vi "LSMcontroller_v63_3Dfocus.vi"() -> ()   [LabVIEW 2015] (continued)
                    n3624 = call "2pparameters.vi"("Params in"=w485, "command"="set") -> ()  [unwired: 1 out]
                  }
                }
              }
            }
          }
          event "Add DO wave": Value Change {
            n3625 = event-data() -> ("NewVal"=w489:bool)  [unwired: 1 in, 5 out]
            n3626 = case shown="True" w489 {
              frame False {
              }
              frame True {
                n3627 = stacked-sequence {
                  seq-local: [_ _ _ _ _ w649 _ _] -> [_ _ _ _ _ _ w664 _]
                  frame #0 {
                    n3628 = local read "Measurement"() -> (w490:T4)
                    n3629 = case shown="\"X-Y-t movie\", Default" w490 {
                      frame "X-Y-t movie", Default {
                        n3630 = local read "avpp"() -> (w511:i32)
                        n3631 = local read "Angle ref"() -> (w510:dbl)
                        n3632 = local read "ROI Type"() -> (w509:u16)
                        n3633 = local read "xpixels ref"() -> (w506:i32)
                        n3634 = local read "Vx-min ref"() -> (w505:dbl)
                        n3635 = local read "Vx-max ref"() -> (w504:dbl)
                        n3636 = local read "ypixels ref"() -> (w502:i32)
                        n3637 = local read "Vy-min ref"() -> (w503:dbl)
                        n3638 = local read "Vy-max ref"() -> (w499:dbl)
                        n3639 = local read "Sampling rate"() -> (w493:dbl)
                        n3640 = local read "finite samples"() -> (w494:bool)
                        n3641 = local read "continuous"() -> (w497:bool)
                        n3642 = local read "wavdet"() -> (w498:bool)
                        n3643 = local read "# of frames"() -> (w496:i32)
                        n3644 = local read "maxbufferAI"() -> (w495:i32)
                        n3645 = local read "Override AI buffer"() -> (w491:bool)
                        n3646 = call "2pparameters.vi"("command"="get") -> ("params out"=w508:T10)  [unwired: 1 in]
                        n3647 = Bundle By Name(cluster=w508, "type"="X-Y-t movie", "avpp"=w511, "Angle Img"=w510, "Xpixels Img"=w506, "Vx-min Img"=w505, "VX-max Img"=w504, "Ypixels Img"=w502, "Vy-min Img"=w503, "Vy-max Img"=w499, "srate"=w493, "srate Img"=w493, "finite"=w494, "cont"=w497, "wavdet"=w498, "measpoints"=w496, "maxbufferAI"=w495, "Drawing Mode"=w509, "Vz-reset"=0.0, "AIoverride"=w491) -> (w500:T10)
                        n3648 = call "2pparameters.vi"("Params in"=w500, "command"="set") -> ()  [unwired: 1 out]
                      }
                      frame "X-Y-Z stack" {
                        n3649 = call "2pparameters.vi"("command"="get") -> ("params out"=w515:T10)  [unwired: 1 in]
                        n3650 = Bundle By Name(cluster=w515, "type"="X-Y-Z stack") -> (w513:T10)
                        n3651 = call "2pparameters.vi"("Params in"=w513, "command"="set") -> ()  [unwired: 1 out]
                      }
                      frame "Lifetime (scan)" {
                        n3652 = call "2pparameters.vi"("command"="get") -> ("params out"=w520:T10)  [unwired: 1 in]
                        n3653 = Bundle By Name(cluster=w520, "type"="Lifetime (scan)") -> (w518:T10)
                        n3654 = call "2pparameters.vi"("Params in"=w518, "command"="set") -> ()  [unwired: 1 out]
                      }
                      frame "Lifetime (contour)" {
                        n3655 = local read "Vy-min draw"() -> (w530:dbl)
                        n3656 = local read "Vy-max draw"() -> (w529:dbl)
                        n3657 = local read "Vx-min draw"() -> (w532:dbl)
                        n3658 = local read "Vx-max draw"() -> (w531:dbl)
                        n3659 = local read "xpixels ref"() -> (w528:i32)
                        n3660 = local read "ypixels ref"() -> (w527:i32)
                        n3661 = local read "ROI Type"() -> (w526:u16)
                        n3662 = local read "srateAODOtt"() -> (w537:dbl)
                        n3663 = local read "# of frames"() -> (w542:i32)
                        n3664 = local read "refreshtime"() -> (w534:dbl)
                        n3665 = local read "Pel"() -> (w525:dbl)
                        n3666 = local read "bin"() -> (w540:dbl)
                        n3667 = local read "Override AI buffer"() -> (w523:bool)
                        n3668 = local read "finite samples"() -> (w549:bool)
                        n3669 = local read "srateAODOtt"() -> (w536:dbl)
                        n3670 = local read "srateAODOtt"() -> (w543:dbl)
                        n3671 = local read "continuous"() -> (w548:bool)
                        n3672 = local read "Angle ref"() -> (w533:dbl)
                        n3673 = local read "wavdet"() -> (w550:bool)
                        n3674 = local read "Vx-ref"() -> (w545:dbl)
                        n3675 = local read "Vy-ref"() -> (w547:dbl)
                        n3676 = local read "avpp"() -> (w546:i32)
                        n3677 = call "tt_timeandsamples.vi"("bin"=w540, "refreshtime"=w534, "srateAODOtt"=w537, "tot#ofsamples"=w542) -> ("refreshrate"=w538:dbl, "refreshbuffer"=w539:i32, "timetracecycles"=w544:i32)  [unwired: 5 in]
                        n3678 = local read "bin"() -> (w541:dbl)
                        n3679 = call "2pparameters.vi"("command"="get") -> ("params out"=w553:T10)  [unwired: 1 in]
                        n3680 = Bundle By Name(cluster=w553, "Drawing Mode"=w526, "measpoints"=w542, "tt_cycles"=w544, "refreshbuffer"=w539, "refreshrate"=w538, "Vx-ref"=w545, "Vy-ref"=w547, "srate"=w536, "finite"=w549, "cont"=w548, "wavdet"=w550, "avpp"=w546, "srateAODO"=w543, "bufferAI"=w539, "bin"=w541, "Angle Img"=w533, "Vxminref"=w532, "Vxmaxref"=w531, "Vyminref"=w530, "Vymaxref"=w529, "Xpixels Img"=w528, "Ypixels Img"=w527, "Pel"=w525, "Vz-reset"=0.0, "AIoverride"=w523, "type"="Lifetime (contour)") -> (w551:T10)
                        n3681 = Reciprocal(x=w538) -> (1/x=w535:dbl)
                        n3682 = local write "refreshtime"(w535) -> ()
                        n3683 = call "2pparameters.vi"("Params in"=w551, "command"="set") -> ()  [unwired: 1 out]
                      }
                      frame "X-Y-Z-t movie" {
                      }
                      frame "linescan" {
                      }
                      frame "Timetrace" {
                        n3684 = local read "Vy-min draw"() -> (w563:dbl)
                        n3685 = local read "Vy-max draw"() -> (w562:dbl)
                        n3686 = local read "Vx-min draw"() -> (w565:dbl)
                        n3687 = local read "Vx-max draw"() -> (w564:dbl)
                        n3688 = local read "xpixels ref"() -> (w561:i32)
                        n3689 = local read "ypixels ref"() -> (w560:i32)
                        n3690 = local read "ROI Type"() -> (w559:u16)
                        n3691 = local read "srateAODOtt"() -> (w570:dbl)
                        n3692 = local read "# of frames"() -> (w575:i32)
                        n3693 = local read "refreshtime"() -> (w567:dbl)
                        n3694 = local read "Pel"() -> (w558:dbl)
                        n3695 = local read "bin"() -> (w573:dbl)
                        n3696 = local read "Override AI buffer"() -> (w556:bool)
                        n3697 = local read "finite samples"() -> (w582:bool)
                        n3698 = local read "srateAODOtt"() -> (w569:dbl)
                        n3699 = local read "srateAODOtt"() -> (w576:dbl)
                        n3700 = local read "continuous"() -> (w581:bool)
                        n3701 = local read "Angle ref"() -> (w566:dbl)
                        n3702 = local read "wavdet"() -> (w583:bool)
                        n3703 = local read "Vx-ref"() -> (w578:dbl)
                        n3704 = local read "Vy-ref"() -> (w580:dbl)
                        n3705 = local read "avpp"() -> (w579:i32)
                        n3706 = call "tt_timeandsamples.vi"("bin"=w573, "refreshtime"=w567, "srateAODOtt"=w570, "tot#ofsamples"=w575) -> ("refreshrate"=w571:dbl, "refreshbuffer"=w572:i32, "timetracecycles"=w577:i32)  [unwired: 5 in]
                        n3707 = local read "bin"() -> (w574:dbl)
                        n3708 = call "2pparameters.vi"("command"="get") -> ("params out"=w586:T10)  [unwired: 1 in]
                        n3709 = Bundle By Name(cluster=w586, "Drawing Mode"=w559, "measpoints"=w575, "tt_cycles"=w577, "refreshbuffer"=w572, "refreshrate"=w571, "Vx-ref"=w578, "Vy-ref"=w580, "srate"=w569, "finite"=w582, "cont"=w581, "wavdet"=w583, "avpp"=w579, "srateAODO"=w576, "bufferAI"=w572, "bin"=w574, "Angle Img"=w566, "Vxminref"=w565, "Vxmaxref"=w564, "Vyminref"=w563, "Vymaxref"=w562, "Xpixels Img"=w561, "Ypixels Img"=w560, "Pel"=w558, "Vz-reset"=0.0, "AIoverride"=w556, "type"="Timetrace") -> (w584:T10)
                        n3710 = Reciprocal(x=w571) -> (1/x=w568:dbl)
                        n3711 = local write "refreshtime"(w568) -> ()
                        n3712 = call "2pparameters.vi"("Params in"=w584, "command"="set") -> ()  [unwired: 1 out]
                      }
                      frame "Lifetime (point)" {
                      }
                    }
                  }
                  frame #1 {
                    w589 = FALSE ("wavdet")
                    n3713 = call "2pparameters.vi"("command"="get") -> ("params out"=w593:T10)  [unwired: 1 in]
                    n3714 = Bundle By Name(cluster=w593, "finite"=w589, "cont"=w589, "wavdet"=TRUE) -> (w590:T10)
                    n3715 = call "2pparameters.vi"("Params in"=w590, "command"="set") -> ()  [unwired: 1 out]
                  }
                  frame #2 {
                    n3716 = local read "DO channels"() -> (w600:u16)
                    n3717 = call "2pparameters.vi"("command"="get") -> ("params out"=w598:T10)  [unwired: 1 in]
                    n3718 = in-place {
                      in-place-border: w600 -> [w604]
                      in-place-border: [w601] -> w595
                      n3719 = in-place-cluster #51(w598) -> ("aDO"=w603:u32[])
                      n3720 = call "add channel to active arrayv2.vi"("line array in"=w603, "line to add"=w604) -> ("line array out"=w602:u32[], "addition"=w601:bool)  [unwired: 1 out]
                      n3721 = in-place-cluster #51("aDO"=w602) -> (w596:T10)
                    }
                    n3722 = local write "addDO"(w595) -> ()
                    n3723 = call "2pparameters.vi"("Params in"=w596, "command"="set") -> ()  [unwired: 1 out]
                  }
                  frame #3 {
                    n3724 = local read "addDO"() -> (w605:bool)
                    n3725 = case shown="True" w605 {
                      frame False {
                      }
                      frame True {
                        n3726 = call "Used AO lines.vi"() -> ("used AO names"=w609:string[], "used AO lines"=w611:tag[])  [unwired: 2 in]
                        n3727 = control-ref of="Analog Lines Plot"() -> (w610:refnum<vi>)
                        n3728 = control-ref of="Digital Lines Plot"() -> (w608:refnum<vi>)
                        n3729 = call "Used DO lines.vi"() -> ("used DO names"=w607:string[], "used DO lines"=w606:tag[])  [unwired: 2 in]
                        n3730 = local write "Analog Used Lines"(w611) -> ()
                        n3731 = local write "Analog Used Names"(w609) -> ()
                        n3732 = local write "Digital Used Lines"(w606) -> ()
                        n3733 = local write "Digital Used Names"(w607) -> ()
                        n3734 = call "prepDOWaveplot.vi"("DigitalGraph in"=w608, "used DO names"=w607) -> ()  [unwired: 1 in]
                        n3735 = call "prepAOWaveplot.vi"("WaveformGraph in"=w610, "Analog Used Names"=w609) -> ()  [unwired: 1 in]
                      }
                    }
                  }
                  frame #4 {
                    n3736 = local read "addDO"() -> (w612:bool)
                    n3737 = case shown="True" w612 {
                      frame False {
                      }
                      frame True {
                        n3738 = local read "Build digital waveform tabs"() -> (w613:enum32{"Simple", "Matlab"})
                        n3739 = case shown="\"Matlab\"" w613 {
                          frame "Simple", Default {
                            n3740 = local read "Meastab"() -> (w615:enum32{"X-Y Image", "Linescan", "Timetrace"})
                            n3741 = call "waveformparamsv2.vi"("command"="get") -> ("Params out"=w629:T14)  [unwired: 4 in, 2 out]
                            n3742 = case shown="\"Timetrace\"" w615 {
                              tunnel: [w631 w632] -> w614
                              frame "X-Y Image", Default {
                                n3743 = local read "Sampling rate"() -> (w631:dbl)
                              }
                              frame "Timetrace" {
                                n3744 = local read "srateAODOtt"() -> (w632:dbl)
                              }
                            }
                            n3745 = Unbundle By Name(w629) -> ("DO parameters"=w627:T17)
                            n3746 = local read "Digital padding value"() -> (w618:dbl)
                            n3747 = local read "Digital time offset (s)"() -> (w619:dbl)
                            n3748 = local read "Digital phase (s)"() -> (w621:dbl)
                            n3749 = local read "Digital Freq (Hz)"() -> (w620:dbl)
                            n3750 = local read "Digital DC (%)"() -> (w622:dbl)
                            n3751 = Index Array(array=w627, index=0) -> (element=w626:T18)
                            n3752 = Bundle By Name(cluster=w626, "Digital DC (%)"=w622, "Digital phase"=w621, "Digital Freq (Hz)"=w620, "Sampling frequency (Hz)"=w614, "Digital time offset (s)"=w619, "padding value"=w618, "matlab wave file"=path "", "DOtab"=0.0) -> (w624:T18)
                            n3753 = Build Array(w624) -> (w623:T17)
                            n3754 = call "waveformparamsv2.vi"("command"="add DO", "add DO"=w623) -> ()  [unwired: 3 in, 3 out]
                          }
                          frame "Matlab" {
                            w636 = 0.0 ("DOtab")
                            n3755 = local read "Meastab"() -> (w634:enum32{"X-Y Image", "Linescan", "Timetrace"})
                            n3756 = call "waveformparamsv2.vi"("command"="get") -> ("Params out"=w645:T14)  [unwired: 4 in, 2 out]
                            n3757 = case shown="\"Timetrace\"" w634 {
                              tunnel: [w647 w648] -> w633
                              frame "X-Y Image", Default {
                                n3758 = local read "Sampling rate"() -> (w647:dbl)
                              }
                              frame "Timetrace" {
                                n3759 = local read "srateAODOtt"() -> (w648:dbl)
                              }
                            }
                            n3760 = Unbundle By Name(w645) -> ("DO parameters"=w643:T17)
                            n3761 = local read "Matlab waveform path DO"() -> (w635:path)
                            n3762 = local read "Matlab padding value DO"() -> (w638:dbl)
                            n3763 = Index Array(array=w643, index=0) -> (element=w642:T18)
                            n3764 = Bundle By Name(cluster=w642, "Digital DC (%)"=w636, "Digital phase"=w636, "Digital Freq (Hz)"=w636, "Sampling frequency (Hz)"=w633, "Digital time offset (s)"=w636, "padding value"=w638, "matlab wave file"=w635, "DOtab"=1.0) -> (w640:T18)
                            n3765 = Build Array(w640) -> (w639:T17)
                            n3766 = call "waveformparamsv2.vi"("command"="add DO", "add DO"=w639) -> ()  [unwired: 3 in, 3 out]
                          }
                        }
                      }
                    }
                  }
                  frame #5 {
                    n3767 = local read "addDO"() -> (w650:bool)
                    n3768 = case shown="True" w650 {
                      tunnel: [_ w651] -> w649
                      frame False {
                      }
                      frame True {
                        n3769 = property on="refwf" class="Ring (strict)"() -> ("RingText.Text"=w656:string)  [unwired: 2 in, 2 out]
                        n3770 = call "waveformsDObuffer.vi"("command"="get") -> ("DO wf out"=w655:digitalwaveform[])  [unwired: 1 in]
                        n3771 = call "waveformsAObuffer.vi"("command"="get") -> ("AO wf out"=w653:waveform(dbl)[])  [unwired: 1 in]
                        n3772 = call "referfencesize.vi"("Digital waveforms in"=w655, "Analog waveforms in"=w653, "reference waveforms to"=w656) -> ("number of samples"=w651:i32)  [unwired: 2 in]
                      }
                    }
                  }
                  frame #6 {
                    n3773 = local read "Build digital waveform tabs"() -> (w667:enum32{"Simple", "Matlab"})
                    n3774 = call "waveformparamsv2.vi"("command"="get last DO") -> ("last DO"=w666:T18)  [unwired: 4 in, 2 out]
                    n3775 = local read "Meastab"() -> (w660:enum32{"X-Y Image", "Linescan", "Timetrace"})
                    n3776 = call "waveformsDObuffer.vi"("command"="get") -> ("DO wf out"=w665:digitalwaveform[])  [unwired: 1 in]
                    n3777 = case shown="\"Simple\", Default" w667 {
                      tunnel: w666 -> [w684 w686]
                      tunnel: w664 -> [w683 _]
                      tunnel: [w682 w685] -> w663
                      frame "Simple", Default {
                        n3778 = call "simple digital from wf params.vi"("waveform params"=w684, "number of samples"=w683) -> ("digital waveform"=w682:digitalwaveform)
                      }
                      frame "Matlab" {
                        n3779 = call "matlabDOwffromparam.vi"("waveform params"=w686) -> ("digital waveform"=w685:digitalwaveform)
                      }
                    }
                    n3780 = property on="refwf" class="Ring (strict)"() -> ("RingText.Text"=w670:string)  [unwired: 2 in, 2 out]
                    n3781 = case shown="\"Timetrace\"" w660 {
                      tunnel: [w679 w680] -> w659
                      frame "X-Y Image", Default {
                        n3782 = local read "Sampling rate"() -> (w679:dbl)
                      }
                      frame "Timetrace" {
                        n3783 = local read "srateAODOtt"() -> (w680:dbl)
                      }
                    }
                    n3784 = call "waveformsAObuffer.vi"("command"="get") -> ("AO wf out"=w678:waveform(dbl)[])  [unwired: 1 in]
                    n3785 = Build Array (concatenate)(w665, w663) -> (w669:digitalwaveform[])
                    n3786 = call "correctwaveformsizetemp.vi"("new sampling frequency (Hz)"=w659, "start"=FALSE, "reference waveforms to"=w670, "Analog waveforms in"=w678, "stop"=FALSE, "Digital waveforms in"=w669) -> ("analog wf out"=w673:waveform(dbl)[], "Digital wf out"=w671:digitalwaveform[], "measpoints"=w661:i32)
                    n3787 = local write "Analog Lines Plot"(w673) -> ()
                    n3788 = call "GetNumCamFramesv2.vi"("Digital Waveform Graph"=w671) -> ("Numeric"=w672:i32)  [unwired: 10 in]
                    n3789 = local write "Digital Lines Plot"(w671) -> ()
                    n3790 = call "waveformsAObuffer.vi"("AO wf in"=w673, "command"="set") -> ()  [unwired: 1 out]
                    n3791 = call "waveformsDObuffer.vi"("DO wf in"=w671, "command"="set") -> ()  [unwired: 1 out]
                    n3792 = local write "Total Camera Frames"(w672) -> ()
                    n3793 = local read "wavdet"() -> (w662:bool)
                    n3794 = case shown="True" w662 {
                      tunnel: w661 -> [_ w681]
                      frame False {
                      }
                      frame True {
                        n3795 = local write "# of frames"(w681) -> ()
                      }
                    }
                  }
                  frame #7 {
                    w687 = FALSE ("addAO")
                    n3796 = local read "finite samples"() -> (w688:bool)
                    n3797 = local read "continuous"() -> (w689:bool)
                    n3798 = local read "wavdet"() -> (w690:bool)
                    n3799 = call "2pparameters.vi"("command"="get") -> ("params out"=w693:T10)  [unwired: 1 in]
                    n3800 = Bundle By Name(cluster=w693, "finite"=w688, "cont"=w689, "wavdet"=w690) -> (w691:T10)
                    n3801 = call "2pparameters.vi"("Params in"=w691, "command"="set") -> ()  [unwired: 1 out]
                    n3802 = local write "addDO"(w687) -> ()
                    n3803 = property on="Add DO wave" class="Bool (strict)"("Val(Sgnl)"=w687) -> ()  [unwired: 2 in, 2 out]
                  }
                }
              }
            }
          }
          event "DO channels": Value Change {
            n3804 = event-data() -> ()  [unwired: 1 in, 6 out]
            n3805 = local read "DO channels"() -> (w697:u16)
            n3806 = call "2pparameters.vi"("command"="get") -> ("params out"=w699:T10)  [unwired: 1 in]
            n3807 = Unbundle By Name(w699) -> ("aDO"=w698:u32[])
            n3808 = Search 1D Array(1D array=w698, element=w697) -> (index of element=w696:i32)  [unwired: 1 in]
            n3809 = Equal?(x=w696, y=-1.0) -> (x = y?=w695:bool)
            n3810 = case shown="False" w695 {
              tunnel: w696 -> [w714 _]
              frame False {
                n3811 = call "waveformparamsv2.vi"("command"="get") -> ("Params out"=w709:T14)  [unwired: 4 in, 2 out]
                n3812 = Unbundle By Name(w709) -> ("DO parameters"=w707:T17)
                n3813 = Index Array(array=w707, index=w714) -> (element=w713:T18)
                n3814 = Unbundle By Name(w713) -> ("Digital DC (%)"=w712:dbl, "Digital phase"=w711:dbl, "Digital Freq (Hz)"=w710:dbl, "Sampling frequency (Hz)"=w702:dbl, "Digital time offset (s)"=w706:dbl, "padding value"=w705:dbl, "matlab wave file"=w704:path, "DOtab"=w703:dbl)
                n3815 = local write "Build digital waveform tabs"(w703) -> ()
                n3816 = local write "Digital DC (%)"(w712) -> ()
                n3817 = local write "Matlab waveform path DO"(w704) -> ()
                n3818 = local write "Digital time offset (s)"(w706) -> ()
                n3819 = local write "Matlab padding value DO"(w705) -> ()
                n3820 = local write "Digital padding value"(w705) -> ()
                n3821 = local write "Sampling rate \ncurrent wf"(w702) -> ()
                n3822 = local write "Digital Freq (Hz)"(w710) -> ()
                n3823 = local write "Digital phase (s)"(w711) -> ()
              }
              frame True {
              }
            }
          }
          event "Rem DO wave": Value Change {
            n3824 = event-data() -> ("NewVal"=w715:bool)  [unwired: 1 in, 5 out]
            n3825 = case shown="True" w715 {
              frame False {
              }
              frame True {
                n3826 = stacked-sequence {
                  seq-local: [_ _ w821 _ _ _ _] -> [_ _ _ _ w840 w851 _]
                  frame #0 {
                    n3827 = local read "Measurement"() -> (w716:T4)
                    n3828 = case shown="\"linescan\"" w716 {
                      frame "X-Y-t movie", Default {
                        n3829 = local read "avpp"() -> (w737:i32)
                        n3830 = local read "Angle ref"() -> (w736:dbl)
                        n3831 = local read "ROI Type"() -> (w735:u16)
                        n3832 = local read "xpixels ref"() -> (w732:i32)
                        n3833 = local read "Vx-min ref"() -> (w731:dbl)
                        n3834 = local read "Vx-max ref"() -> (w730:dbl)
                        n3835 = local read "ypixels ref"() -> (w728:i32)
                        n3836 = local read "Vy-min ref"() -> (w729:dbl)
                        n3837 = local read "Vy-max ref"() -> (w725:dbl)
                        n3838 = local read "Sampling rate"() -> (w719:dbl)
                        n3839 = local read "finite samples"() -> (w720:bool)
                        n3840 = local read "continuous"() -> (w723:bool)
                        n3841 = local read "wavdet"() -> (w724:bool)
                        n3842 = local read "# of frames"() -> (w722:i32)
                        n3843 = local read "maxbufferAI"() -> (w721:i32)
                        n3844 = local read "Override AI buffer"() -> (w717:bool)
                        n3845 = call "2pparameters.vi"("command"="get") -> ("params out"=w734:T10)  [unwired: 1 in]
                        n3846 = Bundle By Name(cluster=w734, "type"="X-Y-t movie", "avpp"=w737, "Angle Img"=w736, "Xpixels Img"=w732, "Vx-min Img"=w731, "VX-max Img"=w730, "Ypixels Img"=w728, "Vy-min Img"=w729, "Vy-max Img"=w725, "srate"=w719, "srate Img"=w719, "finite"=w720, "cont"=w723, "wavdet"=w724, "measpoints"=w722, "maxbufferAI"=w721, "Drawing Mode"=w735, "Vz-reset"=0.0, "AIoverride"=w717) -> (w726:T10)
                        n3847 = call "2pparameters.vi"("Params in"=w726, "command"="set") -> ()  [unwired: 1 out]
                      }
                      frame "X-Y-Z stack" {
                        n3848 = call "2pparameters.vi"("command"="get") -> ("params out"=w741:T10)  [unwired: 1 in]
                        n3849 = Bundle By Name(cluster=w741, "type"="X-Y-Z stack") -> (w739:T10)
                        n3850 = call "2pparameters.vi"("Params in"=w739, "command"="set") -> ()  [unwired: 1 out]
                      }
                      frame "Lifetime (scan)" {
                        n3851 = call "2pparameters.vi"("command"="get") -> ("params out"=w746:T10)  [unwired: 1 in]
                        n3852 = Bundle By Name(cluster=w746, "type"="Lifetime (scan)") -> (w744:T10)
                        n3853 = call "2pparameters.vi"("Params in"=w744, "command"="set") -> ()  [unwired: 1 out]
                      }
                      frame "Lifetime (contour)" {
                        n3854 = local read "Vy-min draw"() -> (w756:dbl)
                        n3855 = local read "Vy-max draw"() -> (w755:dbl)
                        n3856 = local read "Vx-min draw"() -> (w758:dbl)
                        n3857 = local read "Vx-max draw"() -> (w757:dbl)
                        n3858 = local read "xpixels ref"() -> (w754:i32)
                        n3859 = local read "ypixels ref"() -> (w753:i32)
                        n3860 = local read "ROI Type"() -> (w752:u16)
                        n3861 = local read "srateAODOtt"() -> (w763:dbl)
                        n3862 = local read "# of frames"() -> (w768:i32)
                        n3863 = local read "refreshtime"() -> (w760:dbl)
                        n3864 = local read "Pel"() -> (w751:dbl)
                        n3865 = local read "bin"() -> (w766:dbl)
                        n3866 = local read "Override AI buffer"() -> (w749:bool)
                        n3867 = local read "finite samples"() -> (w775:bool)
                        n3868 = local read "srateAODOtt"() -> (w762:dbl)
                        n3869 = local read "srateAODOtt"() -> (w769:dbl)
                        n3870 = local read "continuous"() -> (w774:bool)
                        n3871 = local read "Angle ref"() -> (w759:dbl)
                        n3872 = local read "wavdet"() -> (w776:bool)
                        n3873 = local read "Vx-ref"() -> (w771:dbl)
                        n3874 = local read "Vy-ref"() -> (w773:dbl)
                        n3875 = local read "avpp"() -> (w772:i32)
                        n3876 = call "tt_timeandsamples.vi"("bin"=w766, "refreshtime"=w760, "srateAODOtt"=w763, "tot#ofsamples"=w768) -> ("refreshrate"=w764:dbl, "refreshbuffer"=w765:i32, "timetracecycles"=w770:i32)  [unwired: 5 in]
                        n3877 = local read "bin"() -> (w767:dbl)
                        n3878 = call "2pparameters.vi"("command"="get") -> ("params out"=w779:T10)  [unwired: 1 in]
                        n3879 = Bundle By Name(cluster=w779, "Drawing Mode"=w752, "measpoints"=w768, "tt_cycles"=w770, "refreshbuffer"=w765, "refreshrate"=w764, "Vx-ref"=w771, "Vy-ref"=w773, "srate"=w762, "finite"=w775, "cont"=w774, "wavdet"=w776, "avpp"=w772, "srateAODO"=w769, "bufferAI"=w765, "bin"=w767, "Angle Img"=w759, "Vxminref"=w758, "Vxmaxref"=w757, "Vyminref"=w756, "Vymaxref"=w755, "Xpixels Img"=w754, "Ypixels Img"=w753, "Pel"=w751, "Vz-reset"=0.0, "AIoverride"=w749, "type"="Lifetime (contour)") -> (w777:T10)
                        n3880 = Reciprocal(x=w764) -> (1/x=w761:dbl)
                        n3881 = local write "refreshtime"(w761) -> ()
                        n3882 = call "2pparameters.vi"("Params in"=w777, "command"="set") -> ()  [unwired: 1 out]
                      }
                      frame "X-Y-Z-t movie" {
                      }
                      frame "linescan" {
                      }
                      frame "Timetrace" {
                        n3883 = local read "Vy-min draw"() -> (w789:dbl)
                        n3884 = local read "Vy-max draw"() -> (w788:dbl)
                        n3885 = local read "Vx-min draw"() -> (w791:dbl)
                        n3886 = local read "Vx-max draw"() -> (w790:dbl)
                        n3887 = local read "xpixels ref"() -> (w787:i32)
                        n3888 = local read "ypixels ref"() -> (w786:i32)
                        n3889 = local read "ROI Type"() -> (w785:u16)
                        n3890 = local read "srateAODOtt"() -> (w796:dbl)
                        n3891 = local read "# of frames"() -> (w801:i32)
                        n3892 = local read "refreshtime"() -> (w793:dbl)
                        n3893 = local read "Pel"() -> (w784:dbl)
                        n3894 = local read "bin"() -> (w799:dbl)
                        n3895 = local read "Override AI buffer"() -> (w782:bool)
                        n3896 = local read "finite samples"() -> (w808:bool)
                        n3897 = local read "srateAODOtt"() -> (w795:dbl)
                        n3898 = local read "srateAODOtt"() -> (w802:dbl)
                        n3899 = local read "continuous"() -> (w807:bool)
                        n3900 = local read "Angle ref"() -> (w792:dbl)
                        n3901 = local read "wavdet"() -> (w809:bool)
                        n3902 = local read "Vx-ref"() -> (w804:dbl)
                        n3903 = local read "Vy-ref"() -> (w806:dbl)
                        n3904 = local read "avpp"() -> (w805:i32)
                        n3905 = call "tt_timeandsamples.vi"("bin"=w799, "refreshtime"=w793, "srateAODOtt"=w796, "tot#ofsamples"=w801) -> ("refreshrate"=w797:dbl, "refreshbuffer"=w798:i32, "timetracecycles"=w803:i32)  [unwired: 5 in]
                        n3906 = local read "bin"() -> (w800:dbl)
                        n3907 = call "2pparameters.vi"("command"="get") -> ("params out"=w812:T10)  [unwired: 1 in]
                        n3908 = Bundle By Name(cluster=w812, "Drawing Mode"=w785, "measpoints"=w801, "tt_cycles"=w803, "refreshbuffer"=w798, "refreshrate"=w797, "Vx-ref"=w804, "Vy-ref"=w806, "srate"=w795, "finite"=w808, "cont"=w807, "wavdet"=w809, "avpp"=w805, "srateAODO"=w802, "bufferAI"=w798, "bin"=w800, "Angle Img"=w792, "Vxminref"=w791, "Vxmaxref"=w790, "Vyminref"=w789, "Vymaxref"=w788, "Xpixels Img"=w787, "Ypixels Img"=w786, "Pel"=w784, "Vz-reset"=0.0, "AIoverride"=w782, "type"="Timetrace") -> (w810:T10)
                        n3909 = Reciprocal(x=w797) -> (1/x=w794:dbl)
                        n3910 = local write "refreshtime"(w794) -> ()
                        n3911 = call "2pparameters.vi"("Params in"=w810, "command"="set") -> ()  [unwired: 1 out]
                      }
                      frame "Lifetime (point)" {
                      }
                    }
                  }
                  frame #1 {
                    w815 = FALSE ("wavdet")
                    n3912 = call "2pparameters.vi"("command"="get") -> ("params out"=w819:T10)  [unwired: 1 in]
                    n3913 = Bundle By Name(cluster=w819, "finite"=w815, "cont"=w815, "wavdet"=TRUE) -> (w816:T10)
                    n3914 = call "2pparameters.vi"("Params in"=w816, "command"="set") -> ()  [unwired: 1 out]
                  }
                  frame #2 {
                    n3915 = local read "DO channels"() -> (w827:u16)
                    n3916 = call "2pparameters.vi"("command"="get") -> ("params out"=w825:T10)  [unwired: 1 in]
                    n3917 = in-place {
                      in-place-border: w827 -> [w832]
                      in-place-border: [w829] -> w822
                      in-place-border: [w828] -> w821
                      n3918 = in-place-cluster #52(w825) -> ("aDO"=w831:u32[])
                      n3919 = call "remove channel from active arrayv2.vi"("line array in"=w831, "line to remove"=w832) -> ("line array out"=w830:u32[], "removal"=w829:bool, "index"=w828:i32)
                      n3920 = in-place-cluster #52("aDO"=w830) -> (w823:T10)
                    }
                    n3921 = local write "remDO"(w822) -> ()
                    n3922 = call "2pparameters.vi"("Params in"=w823, "command"="set") -> ()  [unwired: 1 out]
                  }
                  frame #3 {
                    n3923 = local read "remDO"() -> (w833:bool)
                    n3924 = case shown="True" w833 {
                      frame False {
                      }
                      frame True {
                        n3925 = call "Used AO lines.vi"() -> ("used AO names"=w837:string[], "used AO lines"=w839:tag[])  [unwired: 2 in]
                        n3926 = local write "Analog Used Lines"(w839) -> ()
                        n3927 = local write "Analog Used Names"(w837) -> ()
                        n3928 = call "Used DO lines.vi"() -> ("used DO names"=w835:string[], "used DO lines"=w834:tag[])  [unwired: 2 in]
                        n3929 = control-ref of="Analog Lines Plot"() -> (w838:refnum<vi>)
                        n3930 = control-ref of="Digital Lines Plot"() -> (w836:refnum<vi>)
                        n3931 = local write "Digital Used Lines"(w834) -> ()
                        n3932 = local write "Digital Used Names"(w835) -> ()
                        n3933 = call "prepAOWaveplot.vi"("WaveformGraph in"=w838, "Analog Used Names"=w837) -> ()  [unwired: 1 in]
                        n3934 = call "prepDOWaveplot.vi"("DigitalGraph in"=w836, "used DO names"=w835) -> ()  [unwired: 1 in]
                      }
                    }
                  }
                  frame #4 {
                    n3935 = local read "remDO"() -> (w841:bool)
                    n3936 = case shown="True" w841 {
                      tunnel: w840 -> [_ w842]
                      frame False {
                      }
                      frame True {
                        n3937 = call "waveformparamsv2.vi"("command"="rem DO", "index"=w842) -> ()  [unwired: 3 in, 3 out]
                      }
                    }
                  }
                  frame #5 {
                    n3938 = local read "Meastab"() -> (w847:enum32{"X-Y Image", "Linescan", "Timetrace"})
                    n3939 = property on="refwf" class="Ring (strict)"() -> ("RingText.Text"=w854:string)  [unwired: 2 in, 2 out]
                    n3940 = call "waveformsDObuffer.vi"("command"="get") -> ("DO wf out"=w853:digitalwaveform[])  [unwired: 1 in]
                    n3941 = case shown="\"Timetrace\"" w847 {
                      tunnel: [w863 w864] -> w846
                      frame "X-Y Image", Default {
                        n3942 = local read "Sampling rate"() -> (w863:dbl)
                      }
                      frame "Timetrace" {
                        n3943 = local read "srateAODOtt"() -> (w864:dbl)
                      }
                    }
                    n3944 = call "waveformsAObuffer.vi"("command"="get") -> ("AO wf out"=w862:waveform(dbl)[])  [unwired: 1 in]
                    n3945 = Delete From Array(array=w853, length=1, index=w851) -> (array with subset deleted=w850:digitalwaveform[])  [unwired: 1 out]
                    n3946 = call "correctwaveformsizetemp.vi"("new sampling frequency (Hz)"=w846, "start"=FALSE, "reference waveforms to"=w854, "Analog waveforms in"=w862, "stop"=FALSE, "Digital waveforms in"=w850) -> ("analog wf out"=w857:waveform(dbl)[], "Digital wf out"=w855:digitalwaveform[], "measpoints"=w848:i32)
                    n3947 = local read "wavdet"() -> (w849:bool)
                    n3948 = call "waveformsAObuffer.vi"("AO wf in"=w857, "command"="set") -> ()  [unwired: 1 out]
                    n3949 = call "waveformsDObuffer.vi"("DO wf in"=w855, "command"="set") -> ()  [unwired: 1 out]
                    n3950 = local write "Analog Lines Plot"(w857) -> ()
                    n3951 = local write "Digital Lines Plot"(w855) -> ()
                    n3952 = call "GetNumCamFramesv2.vi"("Digital Waveform Graph"=w855) -> ("Numeric"=w856:i32)  [unwired: 10 in]
                    n3953 = case shown="True" w849 {
                      tunnel: w848 -> [_ w865]
                      frame False {
                      }
                      frame True {
                        n3954 = local write "# of frames"(w865) -> ()
                      }
                    }
                    n3955 = local write "Total Camera Frames"(w856) -> ()
                  }
                  frame #6 {
                    w866 = FALSE ("addAO")
                    n3956 = local read "finite samples"() -> (w867:bool)
                    n3957 = local read "continuous"() -> (w868:bool)
                    n3958 = local read "wavdet"() -> (w869:bool)
                    n3959 = local write "remDO"(w866) -> ()
                    n3960 = call "2pparameters.vi"("command"="get") -> ("params out"=w872:T10)  [unwired: 1 in]
                    n3961 = Bundle By Name(cluster=w872, "finite"=w867, "cont"=w868, "wavdet"=w869) -> (w870:T10)
                    n3962 = property on="Rem DO wave" class="Bool (strict)"("Val(Sgnl)"=w866) -> ()  [unwired: 2 in, 2 out]
                    n3963 = call "2pparameters.vi"("Params in"=w870, "command"="set") -> ()  [unwired: 1 out]
                  }
                }
              }
            }
          }
          event "Digital phase (s)", "Digital DC (%)", "Digital Freq (Hz)", "Digital padding value", "Digital time offset (s)": Value Change {
            n3964 = event-data() -> ()  [unwired: 1 in, 6 out]
            n3965 = stacked-sequence {
              seq-local: [_ _ w980 _ _] -> [_ _ _ w997 _]
              seq-local: [_ _ w979 _ _] -> [_ _ _ w996 _]
              frame #0 {
                n3966 = local read "Measurement"() -> (w874:T4)
                n3967 = case shown="\"X-Y-t movie\", Default" w874 {
                  frame "X-Y-t movie", Default {
                    n3968 = local read "avpp"() -> (w895:i32)
                    n3969 = local read "Angle ref"() -> (w894:dbl)
                    n3970 = local read "ROI Type"() -> (w893:u16)
                    n3971 = local read "xpixels ref"() -> (w890:i32)
                    n3972 = local read "Vx-min ref"() -> (w889:dbl)
                    n3973 = local read "Vx-max ref"() -> (w888:dbl)
                    n3974 = local read "ypixels ref"() -> (w886:i32)
                    n3975 = local read "Vy-min ref"() -> (w887:dbl)
                    n3976 = local read "Vy-max ref"() -> (w883:dbl)
                    n3977 = local read "Sampling rate"() -> (w877:dbl)
                    n3978 = local read "finite samples"() -> (w878:bool)
                    n3979 = local read "continuous"() -> (w881:bool)
                    n3980 = local read "wavdet"() -> (w882:bool)
                    n3981 = local read "# of frames"() -> (w880:i32)
                    n3982 = local read "maxbufferAI"() -> (w879:i32)
                    n3983 = local read "Override AI buffer"() -> (w875:bool)
                    n3984 = call "2pparameters.vi"("command"="get") -> ("params out"=w892:T10)  [unwired: 1 in]
                    n3985 = Bundle By Name(cluster=w892, "type"="X-Y-t movie", "avpp"=w895, "Angle Img"=w894, "Xpixels Img"=w890, "Vx-min Img"=w889, "VX-max Img"=w888, "Ypixels Img"=w886, "Vy-min Img"=w887, "Vy-max Img"=w883, "srate"=w877, "srate Img"=w877, "finite"=w878, "cont"=w881, "wavdet"=w882, "measpoints"=w880, "maxbufferAI"=w879, "Drawing Mode"=w893, "Vz-reset"=0.0, "AIoverride"=w875) -> (w884:T10)
                    n3986 = call "2pparameters.vi"("Params in"=w884, "command"="set") -> ()  [unwired: 1 out]
                  }
                  frame "X-Y-Z stack" {
                    n3987 = call "2pparameters.vi"("command"="get") -> ("params out"=w899:T10)  [unwired: 1 in]
                    n3988 = Bundle By Name(cluster=w899, "type"="X-Y-Z stack") -> (w897:T10)
                    n3989 = call "2pparameters.vi"("Params in"=w897, "command"="set") -> ()  [unwired: 1 out]
                  }
                  frame "Lifetime (scan)" {
                    n3990 = call "2pparameters.vi"("command"="get") -> ("params out"=w904:T10)  [unwired: 1 in]
                    n3991 = Bundle By Name(cluster=w904, "type"="Lifetime (scan)") -> (w902:T10)
                    n3992 = call "2pparameters.vi"("Params in"=w902, "command"="set") -> ()  [unwired: 1 out]
                  }
                  frame "Lifetime (contour)" {
                    n3993 = local read "Vy-min draw"() -> (w914:dbl)
                    n3994 = local read "Vy-max draw"() -> (w913:dbl)
                    n3995 = local read "Vx-min draw"() -> (w916:dbl)
                    n3996 = local read "Vx-max draw"() -> (w915:dbl)
                    n3997 = local read "xpixels ref"() -> (w912:i32)
                    n3998 = local read "ypixels ref"() -> (w911:i32)
                    n3999 = local read "ROI Type"() -> (w910:u16)
                    n4000 = local read "srateAODOtt"() -> (w921:dbl)
                    n4001 = local read "# of frames"() -> (w926:i32)
                    n4002 = local read "refreshtime"() -> (w918:dbl)
                    n4003 = local read "Pel"() -> (w909:dbl)
                    n4004 = local read "bin"() -> (w924:dbl)
                    n4005 = local read "Override AI buffer"() -> (w907:bool)
                    n4006 = local read "finite samples"() -> (w933:bool)
                    n4007 = local read "srateAODOtt"() -> (w920:dbl)
                    n4008 = local read "srateAODOtt"() -> (w927:dbl)
                    n4009 = local read "continuous"() -> (w932:bool)
                    n4010 = local read "Angle ref"() -> (w917:dbl)
                    n4011 = local read "wavdet"() -> (w934:bool)
                    n4012 = local read "Vx-ref"() -> (w929:dbl)
                    n4013 = local read "Vy-ref"() -> (w931:dbl)
                    n4014 = local read "avpp"() -> (w930:i32)
                    n4015 = call "tt_timeandsamples.vi"("bin"=w924, "refreshtime"=w918, "srateAODOtt"=w921, "tot#ofsamples"=w926) -> ("refreshrate"=w922:dbl, "refreshbuffer"=w923:i32, "timetracecycles"=w928:i32)  [unwired: 5 in]
                    n4016 = local read "bin"() -> (w925:dbl)
                    n4017 = call "2pparameters.vi"("command"="get") -> ("params out"=w937:T10)  [unwired: 1 in]
                    n4018 = Bundle By Name(cluster=w937, "Drawing Mode"=w910, "measpoints"=w926, "tt_cycles"=w928, "refreshbuffer"=w923, "refreshrate"=w922, "Vx-ref"=w929, "Vy-ref"=w931, "srate"=w920, "finite"=w933, "cont"=w932, "wavdet"=w934, "avpp"=w930, "srateAODO"=w927, "bufferAI"=w923, "bin"=w925, "Angle Img"=w917, "Vxminref"=w916, "Vxmaxref"=w915, "Vyminref"=w914, "Vymaxref"=w913, "Xpixels Img"=w912, "Ypixels Img"=w911, "Pel"=w909, "Vz-reset"=0.0, "AIoverride"=w907, "type"="Lifetime (contour)") -> (w935:T10)
                    n4019 = Reciprocal(x=w922) -> (1/x=w919:dbl)
                    n4020 = local write "refreshtime"(w919) -> ()
                    n4021 = call "2pparameters.vi"("Params in"=w935, "command"="set") -> ()  [unwired: 1 out]
                  }
                  frame "X-Y-Z-t movie" {
                  }
                  frame "linescan" {
                  }
                  frame "Timetrace" {
                    n4022 = local read "Vy-min draw"() -> (w947:dbl)
                    n4023 = local read "Vy-max draw"() -> (w946:dbl)
                    n4024 = local read "Vx-min draw"() -> (w949:dbl)
                    n4025 = local read "Vx-max draw"() -> (w948:dbl)
                    n4026 = local read "xpixels ref"() -> (w945:i32)
                    n4027 = local read "ypixels ref"() -> (w944:i32)
                    n4028 = local read "ROI Type"() -> (w943:u16)
                    n4029 = local read "srateAODOtt"() -> (w954:dbl)
                    n4030 = local read "# of frames"() -> (w959:i32)
                    n4031 = local read "refreshtime"() -> (w951:dbl)
                    n4032 = local read "Pel"() -> (w942:dbl)
                    n4033 = local read "bin"() -> (w957:dbl)
                    n4034 = local read "Override AI buffer"() -> (w940:bool)
                    n4035 = local read "finite samples"() -> (w966:bool)
                    n4036 = local read "srateAODOtt"() -> (w953:dbl)
                    n4037 = local read "srateAODOtt"() -> (w960:dbl)
                    n4038 = local read "continuous"() -> (w965:bool)
                    n4039 = local read "Angle ref"() -> (w950:dbl)
                    n4040 = local read "wavdet"() -> (w967:bool)
                    n4041 = local read "Vx-ref"() -> (w962:dbl)
                    n4042 = local read "Vy-ref"() -> (w964:dbl)
                    n4043 = local read "avpp"() -> (w963:i32)
                    n4044 = call "tt_timeandsamples.vi"("bin"=w957, "refreshtime"=w951, "srateAODOtt"=w954, "tot#ofsamples"=w959) -> ("refreshrate"=w955:dbl, "refreshbuffer"=w956:i32, "timetracecycles"=w961:i32)  [unwired: 5 in]
                    n4045 = local read "bin"() -> (w958:dbl)
                    n4046 = call "2pparameters.vi"("command"="get") -> ("params out"=w970:T10)  [unwired: 1 in]
                    n4047 = Bundle By Name(cluster=w970, "Drawing Mode"=w943, "measpoints"=w959, "tt_cycles"=w961, "refreshbuffer"=w956, "refreshrate"=w955, "Vx-ref"=w962, "Vy-ref"=w964, "srate"=w953, "finite"=w966, "cont"=w965, "wavdet"=w967, "avpp"=w963, "srateAODO"=w960, "bufferAI"=w956, "bin"=w958, "Angle Img"=w950, "Vxminref"=w949, "Vxmaxref"=w948, "Vyminref"=w947, "Vymaxref"=w946, "Xpixels Img"=w945, "Ypixels Img"=w944, "Pel"=w942, "Vz-reset"=0.0, "AIoverride"=w940, "type"="Timetrace") -> (w968:T10)
                    n4048 = Reciprocal(x=w955) -> (1/x=w952:dbl)
                    n4049 = local write "refreshtime"(w952) -> ()
                    n4050 = call "2pparameters.vi"("Params in"=w968, "command"="set") -> ()  [unwired: 1 out]
                  }
                  frame "Lifetime (point)" {
                  }
                }
              }
              frame #1 {
                w973 = FALSE ("wavdet")
                n4051 = call "2pparameters.vi"("command"="get") -> ("params out"=w977:T10)  [unwired: 1 in]
                n4052 = Bundle By Name(cluster=w977, "finite"=w973, "cont"=w973, "wavdet"=TRUE) -> (w974:T10)
                n4053 = call "2pparameters.vi"("Params in"=w974, "command"="set") -> ()  [unwired: 1 out]
              }
              frame #2 {
                n4054 = local read "DO channels"() -> (w982:u16)
                n4055 = call "2pparameters.vi"("command"="get") -> ("params out"=w984:T10)  [unwired: 1 in]
                n4056 = Unbundle By Name(w984) -> ("aDO"=w983:u32[])
                n4057 = Search 1D Array(1D array=w983, element=w982) -> (index of element=w980:i32)  [unwired: 1 in]
                n4058 = Greater?(x=w980, y=-1) -> (0:w979:bool)
                n4059 = case shown="True" w979 {
                  tunnel: w980 -> [_ w993]
                  frame False {
                  }
                  frame True {
                    n4060 = local read "Meastab"() -> (w987:enum32{"X-Y Image", "Linescan", "Timetrace"})
                    n4061 = local read "Digital padding value"() -> (w988:dbl)
                    n4062 = local read "Digital time offset (s)"() -> (w989:dbl)
                    n4063 = case shown="\"Timetrace\"" w987 {
                      tunnel: [w994 w995] -> w986
                      frame "X-Y Image", Default {
                        n4064 = local read "Sampling rate"() -> (w994:dbl)
                      }
                      frame "Timetrace" {
                        n4065 = local read "srateAODOtt"() -> (w995:dbl)
                      }
                    }
                    n4066 = local read "Digital Freq (Hz)"() -> (w991:dbl)
                    n4067 = local read "Digital phase (s)"() -> (w990:dbl)
                    n4068 = local read "Digital DC (%)"() -> (w992:dbl)
                    n4069 = call "replace DO wf param.vi"("Digital Freq (Hz)"=w991, "Digital DC (%)"=w992, "Digital phase"=w990, "Sampling frequency (Hz)"=w986, "Digital time offset (s)"=w989, "index of DO wave"=w993, "padding value"=w988) -> ()  [unwired: 4 in]
                  }
                }
              }
              frame #3 {
                n4070 = case shown="True" w996 {
                  tunnel: w997 -> [_ w1004]
                  frame False {
                  }
                  frame True {
                    n4071 = local read "Meastab"() -> (w1001:enum32{"X-Y Image", "Linescan", "Timetrace"})
                    n4072 = call "waveformparamsv2.vi"("command"="get") -> ("Params out"=w1020:T14)  [unwired: 4 in, 2 out]
                    n4073 = Unbundle By Name(w1020) -> ("DO parameters"=w1019:T17)
                    n4074 = property on="refwf" class="Ring (strict)"() -> ("RingText.Text"=w1026:string)  [unwired: 2 in, 2 out]
                    n4075 = case shown="\"Timetrace\"" w1001 {
                      tunnel: [w1027 w1028] -> w1000
                      frame "X-Y Image", Default {
                        n4076 = local read "Sampling rate"() -> (w1027:dbl)
                      }
                      frame "Timetrace" {
                        n4077 = local read "srateAODOtt"() -> (w1028:dbl)
                      }
                    }
                    n4078 = call "waveformsAObuffer.vi"("command"="get") -> ("AO wf out"=w1024:waveform(dbl)[])  [unwired: 1 in]
                    n4079 = call "waveformsDObuffer.vi"("command"="get") -> ("DO wf out"=w1022:digitalwaveform[])  [unwired: 1 in]
                    n4080 = call "referfencesize.vi"("Digital waveforms in"=w1022, "Analog waveforms in"=w1024, "reference waveforms to"=w1026) -> ("number of samples"=w1017:i32)  [unwired: 2 in]
                    n4081 = Index Array(array=w1019, index=w1004) -> (element=w1018:T18)
                    n4082 = call "waveformsDObuffer.vi"("command"="get") -> ("DO wf out"=w1014:digitalwaveform[])  [unwired: 1 in]
                    n4083 = call "simple digital from wf params.vi"("waveform params"=w1018, "number of samples"=w1017) -> ("digital waveform"=w1016:digitalwaveform)
                    n4084 = property on="refwf" class="Ring (strict)"() -> ("RingText.Text"=w1006:string)  [unwired: 2 in, 2 out]
                    n4085 = Replace Array Subset(array=w1014, new element=w1016, index=w1004) -> (w1005:digitalwaveform[])
                    n4086 = call "waveformsAObuffer.vi"("command"="get") -> ("AO wf out"=w1013:waveform(dbl)[])  [unwired: 1 in]
                    n4087 = local read "wavdet"() -> (w1003:bool)
                    n4088 = call "correctwaveformsizetemp.vi"("new sampling frequency (Hz)"=w1000, "start"=FALSE, "reference waveforms to"=w1006, "Analog waveforms in"=w1013, "stop"=FALSE, "Digital waveforms in"=w1005) -> ("analog wf out"=w1009:waveform(dbl)[], "Digital wf out"=w1007:digitalwaveform[], "measpoints"=w1002:i32)
                    n4089 = local write "Analog Lines Plot"(w1009) -> ()
                    n4090 = call "GetNumCamFramesv2.vi"("Digital Waveform Graph"=w1007) -> ("Numeric"=w1008:i32)  [unwired: 10 in]
                    n4091 = local write "Digital Lines Plot"(w1007) -> ()
                    n4092 = case shown="True" w1003 {
                      tunnel: w1002 -> [_ w1029]
                      frame False {
                      }
                      frame True {
                        n4093 = local write "# of frames"(w1029) -> ()
                      }
                    }
                    n4094 = call "waveformsAObuffer.vi"("AO wf in"=w1009, "command"="set") -> ()  [unwired: 1 out]
                    n4095 = call "waveformsDObuffer.vi"("DO wf in"=w1007, "command"="set") -> ()  [unwired: 1 out]
                    n4096 = local write "Total Camera Frames"(w1008) -> ()
                  }
                }
              }
              frame #4 {
                n4097 = local read "finite samples"() -> (w1030:bool)
                n4098 = local read "continuous"() -> (w1031:bool)
                n4099 = local read "wavdet"() -> (w1032:bool)
                n4100 = call "2pparameters.vi"("command"="get") -> ("params out"=w1035:T10)  [unwired: 1 in]
                n4101 = Bundle By Name(cluster=w1035, "finite"=w1030, "cont"=w1031, "wavdet"=w1032) -> (w1033:T10)
                n4102 = call "2pparameters.vi"("Params in"=w1033, "command"="set") -> ()  [unwired: 1 out]
              }
            }
          }
          event "refwf": Value Change {
            n4103 = event-data() -> ()  [unwired: 1 in, 6 out]
            n4104 = stacked-sequence {
              frame #0 {
                n4105 = local read "Measurement"() -> (w1037:T4)
                n4106 = case shown="\"X-Y-t movie\", Default" w1037 {
                  frame "X-Y-t movie", Default {
                    n4107 = local read "avpp"() -> (w1058:i32)
                    n4108 = local read "Angle ref"() -> (w1057:dbl)
                    n4109 = local read "ROI Type"() -> (w1056:u16)
                    n4110 = local read "xpixels ref"() -> (w1053:i32)
                    n4111 = local read "Vx-min ref"() -> (w1052:dbl)
                    n4112 = local read "Vx-max ref"() -> (w1051:dbl)
                    n4113 = local read "ypixels ref"() -> (w1049:i32)
                    n4114 = local read "Vy-min ref"() -> (w1050:dbl)
                    n4115 = local read "Vy-max ref"() -> (w1046:dbl)
                    n4116 = local read "Sampling rate"() -> (w1040:dbl)
                    n4117 = local read "finite samples"() -> (w1041:bool)
                    n4118 = local read "continuous"() -> (w1044:bool)
                    n4119 = local read "wavdet"() -> (w1045:bool)
                    n4120 = local read "# of frames"() -> (w1043:i32)
                    n4121 = local read "maxbufferAI"() -> (w1042:i32)
                    n4122 = local read "Override AI buffer"() -> (w1038:bool)
                    n4123 = call "2pparameters.vi"("command"="get") -> ("params out"=w1055:T10)  [unwired: 1 in]
                    n4124 = Bundle By Name(cluster=w1055, "type"="X-Y-t movie", "avpp"=w1058, "Angle Img"=w1057, "Xpixels Img"=w1053, "Vx-min Img"=w1052, "VX-max Img"=w1051, "Ypixels Img"=w1049, "Vy-min Img"=w1050, "Vy-max Img"=w1046, "srate"=w1040, "srate Img"=w1040, "finite"=w1041, "cont"=w1044, "wavdet"=w1045, "measpoints"=w1043, "maxbufferAI"=w1042, "Drawing Mode"=w1056, "Vz-reset"=0.0, "AIoverride"=w1038) -> (w1047:T10)
                    n4125 = call "2pparameters.vi"("Params in"=w1047, "command"="set") -> ()  [unwired: 1 out]
                  }
                  frame "X-Y-Z stack" {
                    n4126 = call "2pparameters.vi"("command"="get") -> ("params out"=w1062:T10)  [unwired: 1 in]
                    n4127 = Bundle By Name(cluster=w1062, "type"="X-Y-Z stack") -> (w1060:T10)
                    n4128 = call "2pparameters.vi"("Params in"=w1060, "command"="set") -> ()  [unwired: 1 out]
                  }
                  frame "Lifetime (scan)" {
                    n4129 = call "2pparameters.vi"("command"="get") -> ("params out"=w1067:T10)  [unwired: 1 in]
                    n4130 = Bundle By Name(cluster=w1067, "type"="Lifetime (scan)") -> (w1065:T10)
                    n4131 = call "2pparameters.vi"("Params in"=w1065, "command"="set") -> ()  [unwired: 1 out]
                  }
                  frame "Lifetime (contour)" {
                    n4132 = local read "Vy-min draw"() -> (w1077:dbl)
                    n4133 = local read "Vy-max draw"() -> (w1076:dbl)
                    n4134 = local read "Vx-min draw"() -> (w1079:dbl)
                    n4135 = local read "Vx-max draw"() -> (w1078:dbl)
                    n4136 = local read "xpixels ref"() -> (w1075:i32)
                    n4137 = local read "ypixels ref"() -> (w1074:i32)
                    n4138 = local read "ROI Type"() -> (w1073:u16)
                    n4139 = local read "srateAODOtt"() -> (w1084:dbl)
                    n4140 = local read "# of frames"() -> (w1089:i32)
                    n4141 = local read "refreshtime"() -> (w1081:dbl)
                    n4142 = local read "Pel"() -> (w1072:dbl)
                    n4143 = local read "bin"() -> (w1087:dbl)
                    n4144 = local read "Override AI buffer"() -> (w1070:bool)
                    n4145 = local read "finite samples"() -> (w1096:bool)
                    n4146 = local read "srateAODOtt"() -> (w1083:dbl)
                    n4147 = local read "srateAODOtt"() -> (w1090:dbl)
                    n4148 = local read "continuous"() -> (w1095:bool)
                    n4149 = local read "Angle ref"() -> (w1080:dbl)
                    n4150 = local read "wavdet"() -> (w1097:bool)
                    n4151 = local read "Vx-ref"() -> (w1092:dbl)
                    n4152 = local read "Vy-ref"() -> (w1094:dbl)
                    n4153 = local read "avpp"() -> (w1093:i32)
                    n4154 = call "tt_timeandsamples.vi"("bin"=w1087, "refreshtime"=w1081, "srateAODOtt"=w1084, "tot#ofsamples"=w1089) -> ("refreshrate"=w1085:dbl, "refreshbuffer"=w1086:i32, "timetracecycles"=w1091:i32)  [unwired: 5 in]
                    n4155 = local read "bin"() -> (w1088:dbl)
                    n4156 = call "2pparameters.vi"("command"="get") -> ("params out"=w1100:T10)  [unwired: 1 in]
                    n4157 = Bundle By Name(cluster=w1100, "Drawing Mode"=w1073, "measpoints"=w1089, "tt_cycles"=w1091, "refreshbuffer"=w1086, "refreshrate"=w1085, "Vx-ref"=w1092, "Vy-ref"=w1094, "srate"=w1083, "finite"=w1096, "cont"=w1095, "wavdet"=w1097, "avpp"=w1093, "srateAODO"=w1090, "bufferAI"=w1086, "bin"=w1088, "Angle Img"=w1080, "Vxminref"=w1079, "Vxmaxref"=w1078, "Vyminref"=w1077, "Vymaxref"=w1076, "Xpixels Img"=w1075, "Ypixels Img"=w1074, "Pel"=w1072, "Vz-reset"=0.0, "AIoverride"=w1070, "type"="Lifetime (contour)") -> (w1098:T10)
                    n4158 = Reciprocal(x=w1085) -> (1/x=w1082:dbl)
                    n4159 = local write "refreshtime"(w1082) -> ()
                    n4160 = call "2pparameters.vi"("Params in"=w1098, "command"="set") -> ()  [unwired: 1 out]
                  }
                  frame "X-Y-Z-t movie" {
                  }
                  frame "linescan" {
                  }
                  frame "Timetrace" {
                    n4161 = local read "Vy-min draw"() -> (w1110:dbl)
                    n4162 = local read "Vy-max draw"() -> (w1109:dbl)
                    n4163 = local read "Vx-min draw"() -> (w1112:dbl)
                    n4164 = local read "Vx-max draw"() -> (w1111:dbl)
                    n4165 = local read "xpixels ref"() -> (w1108:i32)
                    n4166 = local read "ypixels ref"() -> (w1107:i32)
                    n4167 = local read "ROI Type"() -> (w1106:u16)
                    n4168 = local read "srateAODOtt"() -> (w1117:dbl)
                    n4169 = local read "# of frames"() -> (w1122:i32)
                    n4170 = local read "refreshtime"() -> (w1114:dbl)
                    n4171 = local read "Pel"() -> (w1105:dbl)
                    n4172 = local read "bin"() -> (w1120:dbl)
                    n4173 = local read "Override AI buffer"() -> (w1103:bool)
                    n4174 = local read "finite samples"() -> (w1129:bool)
                    n4175 = local read "srateAODOtt"() -> (w1116:dbl)
                    n4176 = local read "srateAODOtt"() -> (w1123:dbl)
                    n4177 = local read "continuous"() -> (w1128:bool)
                    n4178 = local read "Angle ref"() -> (w1113:dbl)
                    n4179 = local read "wavdet"() -> (w1130:bool)
                    n4180 = local read "Vx-ref"() -> (w1125:dbl)
                    n4181 = local read "Vy-ref"() -> (w1127:dbl)
                    n4182 = local read "avpp"() -> (w1126:i32)
                    n4183 = call "tt_timeandsamples.vi"("bin"=w1120, "refreshtime"=w1114, "srateAODOtt"=w1117, "tot#ofsamples"=w1122) -> ("refreshrate"=w1118:dbl, "refreshbuffer"=w1119:i32, "timetracecycles"=w1124:i32)  [unwired: 5 in]
                    n4184 = local read "bin"() -> (w1121:dbl)
                    n4185 = call "2pparameters.vi"("command"="get") -> ("params out"=w1133:T10)  [unwired: 1 in]
                    n4186 = Bundle By Name(cluster=w1133, "Drawing Mode"=w1106, "measpoints"=w1122, "tt_cycles"=w1124, "refreshbuffer"=w1119, "refreshrate"=w1118, "Vx-ref"=w1125, "Vy-ref"=w1127, "srate"=w1116, "finite"=w1129, "cont"=w1128, "wavdet"=w1130, "avpp"=w1126, "srateAODO"=w1123, "bufferAI"=w1119, "bin"=w1121, "Angle Img"=w1113, "Vxminref"=w1112, "Vxmaxref"=w1111, "Vyminref"=w1110, "Vymaxref"=w1109, "Xpixels Img"=w1108, "Ypixels Img"=w1107, "Pel"=w1105, "Vz-reset"=0.0, "AIoverride"=w1103, "type"="Timetrace") -> (w1131:T10)
                    n4187 = Reciprocal(x=w1118) -> (1/x=w1115:dbl)
                    n4188 = local write "refreshtime"(w1115) -> ()
                    n4189 = call "2pparameters.vi"("Params in"=w1131, "command"="set") -> ()  [unwired: 1 out]
                  }
                  frame "Lifetime (point)" {
                  }
                }
              }
              frame #1 {
                w1136 = FALSE ("wavdet")
                n4190 = call "2pparameters.vi"("command"="get") -> ("params out"=w1140:T10)  [unwired: 1 in]
                n4191 = Bundle By Name(cluster=w1140, "finite"=w1136, "cont"=w1136, "wavdet"=TRUE) -> (w1137:T10)
                n4192 = call "2pparameters.vi"("Params in"=w1137, "command"="set") -> ()  [unwired: 1 out]
              }
              frame #2 {
                n4193 = local read "Meastab"() -> (w1145:enum32{"X-Y Image", "Linescan", "Timetrace"})
                n4194 = property on="refwf" class="Ring (strict)"() -> ("RingText.Text"=w1148:string)  [unwired: 2 in, 2 out]
                n4195 = case shown="\"Timetrace\"" w1145 {
                  tunnel: [w1158 w1159] -> w1144
                  frame "X-Y Image", Default {
                    n4196 = local read "Sampling rate"() -> (w1158:dbl)
                  }
                  frame "Timetrace" {
                    n4197 = local read "srateAODOtt"() -> (w1159:dbl)
                  }
                }
